vi "target.vi"() -> ()   [LabVIEW 2020]
uses:
  <vilib>/rvi/interface/RandomDataEmulation/niFpgaRandomDataHandleErrors.vi
  <vilib>/ARTS-Lab/Array-based Linear Algebra/matrix_matrix_VIs/matrix_matrix_multiply_SGL.vi
  <vilib>/rvi/DataTransferAndStorage/Container/XNode/niFpgaContainer.xnode
  <vilib>/rvi/interface/RandomDataEmulation/nirviRandomDataFpgaReadWriteTemplate.vi
panel:
  out "ticks":u32
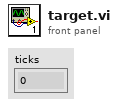
[diagram p1: front panel]
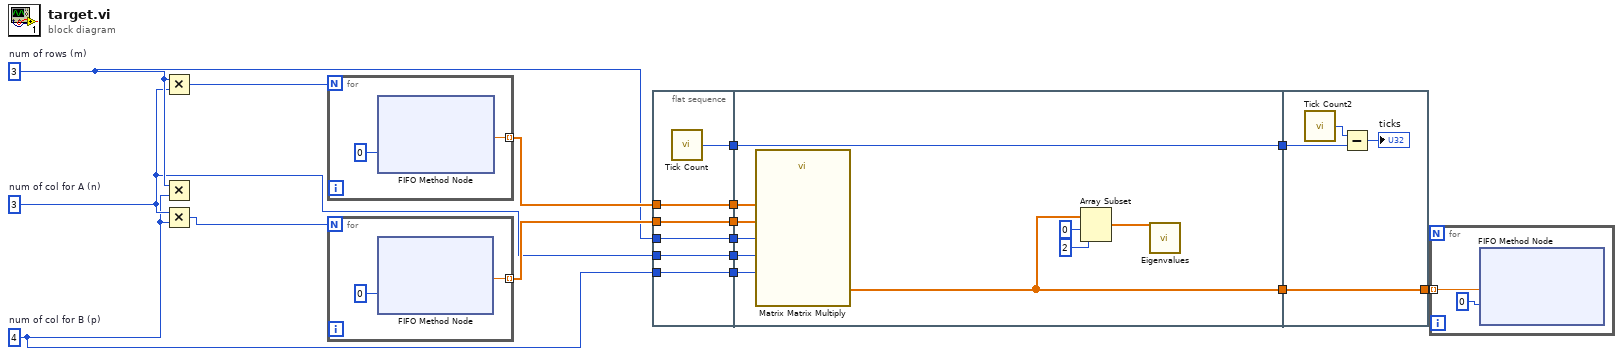
[diagram p0: block diagram]
diagram:
  w10 = 4  # num of col for B (p)
  w11 = 3  # num of col for A (n)
  w12 = 3  # num of rows (m)
  n1 = Multiply(x=w12, y=w11) -> (x*y=w16:i32)
  n2 = Multiply(x=w12, y=w10) -> ()  [unwired: 1 out]
  n3 = Multiply(x=w11, y=w10) -> (x*y=w15:i32)
  n4 = for {
    N: w16 -> [_]
    tunnel: [w18] -> w14 mode=indexing
    n5 = xnode ("FIFO Method Node")("Timeout"=0) -> ("Element"=w18:sgl)  [unwired: 1 in, 2 out]
  }
  n6 = for {
    N: w15 -> [_]
    tunnel: [w19] -> w13 mode=indexing
    n7 = xnode ("FIFO Method Node")("Timeout"=0) -> ("Element"=w19:sgl)  [unwired: 1 in, 2 out]
  }
  n8 = flat-sequence {
    tunnel: w10 -> [w22]
    tunnel: w11 -> [w23]
    tunnel: w12 -> [w24]
    tunnel: w13 -> [w25]
    tunnel: w14 -> [w26]
    tunnel: [w26] -> w8
    tunnel: [w25] -> w7
    tunnel: [w24] -> w6
    tunnel: [w23] -> w5
    tunnel: [w22] -> w4
    tunnel: [w21] -> w2
    tunnel: w8 -> [w36]
    tunnel: w7 -> [w35]
    tunnel: w6 -> [w34]
    tunnel: w5 -> [w33]
    tunnel: w4 -> [w32]
    tunnel: [w30] -> w3
    tunnel: w2 -> [w31]
    tunnel: [w31] -> w1
    tunnel: [w40] -> w9
    tunnel: w3 -> [w40]
    tunnel: w1 -> [w38]
    frame #0 {
      n9 = call "Tick Count"() -> ("Tick Count(Ticks)"=w21:u32)
    }
    frame #1 {
      n10 = call-poly <vilib>:"Matrix Matrix Multiply.vi"("p"=w32, "n"=w33, "m"=w34, "B"=w35, "A"=w36) -> ("C"=w30:sgl[])  [unwired: 1 in]
      n11 = Array Subset(array=w30, index=0, length=2) -> (w27:sgl[])
      n12 = call <vilib>:"Eigenvalues.vi"("A"=w27) -> ()  [unwired: 2 in, 1 out]
    }
    frame #2 {
      n13 = call "Tick Count2"() -> ("Tick Count(Ticks)"=w39:u32)
      n14 = Subtract(x=w39, y=w38) -> (x-y=→"ticks":u32)
    }
  }
  n15 = for {
    tunnel: w9 -> [w42] mode=indexing
    n16 = xnode ("FIFO Method Node")("Element"=w42, "Timeout"=0) -> ()  [unwired: 1 in, 2 out]
  }
